vi "Format InstanceNetworkInterfaceSetItemType_LVXML_Loop.vi"(8 "error in (no error)":errorcluster, 10 "Siblings in 3":T2(array[cluster]), 11 "AWS_EC2 in":refnum<class "AWS_EC2.lvclass">) -> (0 "error out":errorcluster, 2 "Array":T3[](array[typedef]), 3 "AWS_EC2 out":refnum<class "AWS_EC2.lvclass">)   [LabVIEW 2014, in "AWS_EC2.lvlib" / "AWS_EC2.lvclass"]
uses:
  AWS_EC2.lvclass
  EC2 Datatypes/InstanceNetworkInterfaceSetItemType.ctl
  EC2 Datatypes/GroupItemTypeSet.ctl
  EC2 Datatypes/GroupItemType.ctl
  EC2 Datatypes/InstanceNetworkInterfaceAttachmentType.ctl
  EC2 Datatypes/InstanceNetworkInterfaceAssociationType.ctl
  EC2 Datatypes/InstancePrivateIpAddressesSetItemType.ctl
  lv-xml-parser/r0/trunk/VI Source/EventType.ctl
  AWS_EC2.lvlib
  lv-xml-parser/r0/trunk/VI Source/LV XML Parser.lvlib
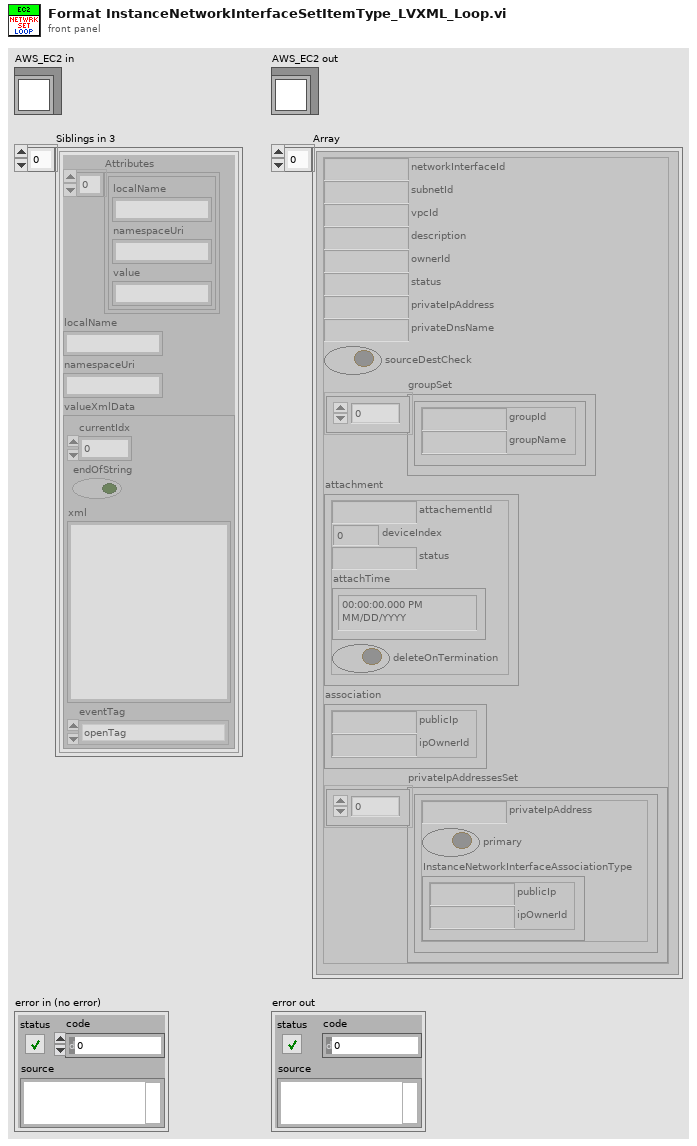
[diagram p1: front panel]
types:
  T1 = typedef "LV XML Parser.lvlib/EventType.ctl" = enum16{"openTag", "endOpenTag", "closeTag", "comment", "endComment", "endOfFile", "attribute", "startXml", "selfClosingTag"}
  T2 = cluster{"Attributes":cluster{"localName":string, "namespaceUri":string, "value":string}[], "localName":string, "namespaceUri":string, "valueXmlData":cluster{"currentIdx":i32, "endOfString":bool, "xml":string, "eventTag":T1}}[]
  T3 = typedef "AWS_EC2.lvlib/InstanceNetworkInterfaceSetItemType.ctl" = cluster{"networkInterfaceId":string, "subnetId":string, "vpcId":string, "description":string, "ownerId":string, "status":string, "privateIpAddress":string, "privateDnsName":string, "sourceDestCheck":bool, "groupSet":T4, "attachment":T6, "association":T7, "privateIpAddressesSet":T8[]}
  T4 = typedef "AWS_EC2.lvlib/GroupItemTypeSet.ctl" = T5[]
  T5 = typedef "AWS_EC2.lvlib/GroupItemType.ctl" = cluster{"groupId":string, "groupName":string}
  T6 = typedef "AWS_EC2.lvlib/InstanceNetworkInterfaceAttachmentType.ctl" = cluster{"attachementId":string, "deviceIndex":i32, "status":string, "attachTime":timestamp, "deleteOnTermination":bool}
  T7 = typedef "AWS_EC2.lvlib/InstanceNetworkInterfaceAssociationType.ctl" = cluster{"publicIp":string, "ipOwnerId":string}
  T8 = typedef "AWS_EC2.lvlib/InstancePrivateIpAddressesSetItemType.ctl" = cluster{"privateIpAddress":string, "primary":bool, "InstanceNetworkInterfaceAssociationType":T7}
  T9 = cluster{"Attributes":cluster{"localName":string, "namespaceUri":string, "value":string}[], "localName":string, "namespaceUri":string, "valueXmlData":cluster{"currentIdx":i32, "endOfString":bool, "xml":string, "eventTag":T1}}
  T10 = cluster{"currentIdx":i32, "endOfString":bool, "xml":string, "eventTag":T1}
  T11 = cluster{"namespaceUri":string, "localName":string}
  T12 = cluster{"Attributes":cluster{"localName":string, "namespaceUri":string, "value":string}[], "localName":string, "namespaceUri":string, "valueXmlData":cluster{"currentIdx":i64, "endOfString":bool, "xml":string, "eventTag":T1}}[]
  T13 = cluster{"currentIdx":i64, "endOfString":bool, "xml":string, "eventTag":T1}
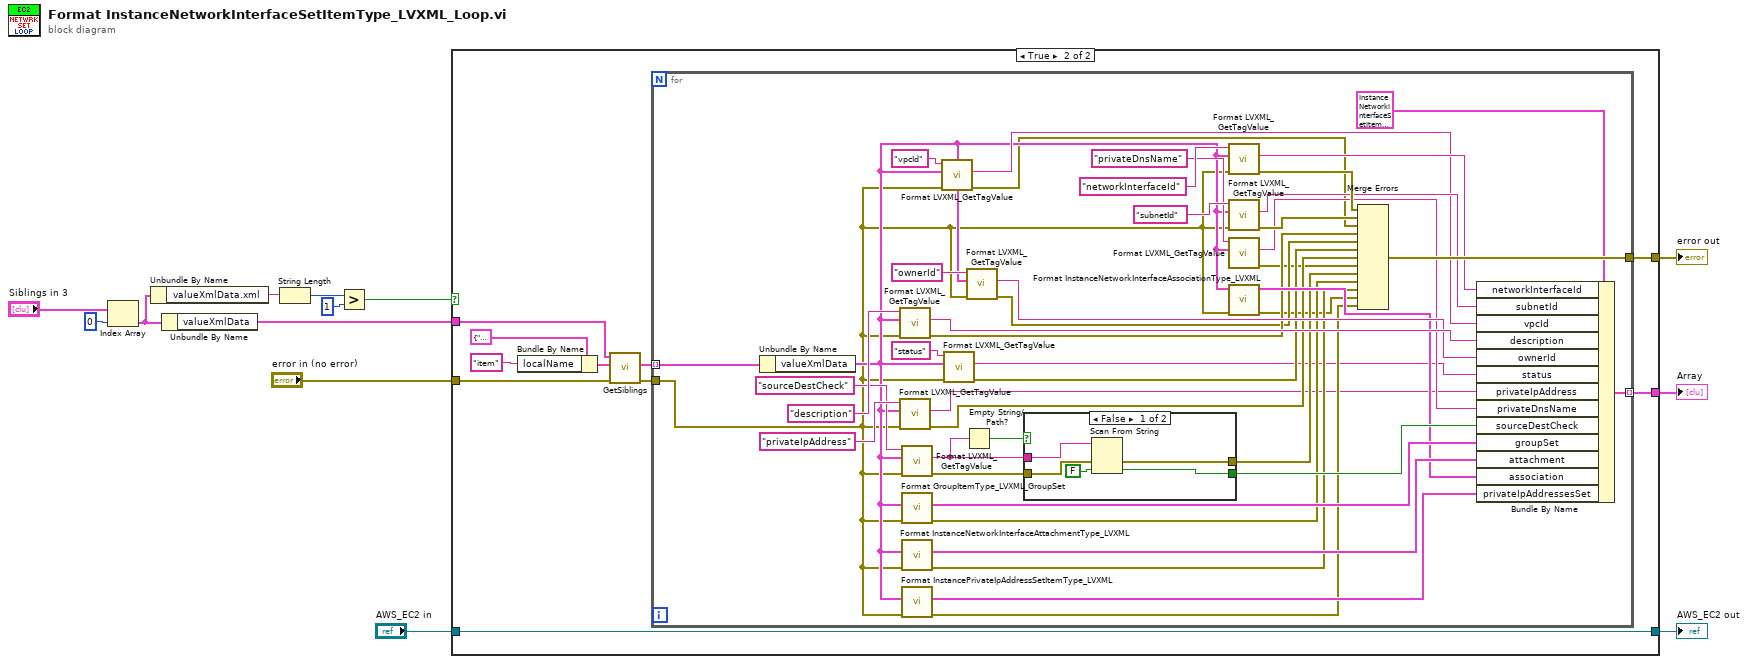
[diagram p0: block diagram]
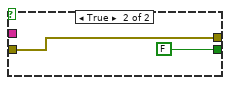
[diagram p3: hidden frame]
diagram:
  n1 = Index Array(array="Siblings in 3", index=0) -> (element=w3:T9)
  n2 = Unbundle By Name(w3) -> ("valueXmlData.xml"=w4:string)
  n3 = Unbundle By Name(w3) -> ("valueXmlData"=w5:T10)
  n4 = String Length(string=w4) -> (length=w8:i32)
  n5 = Greater?(x=w8, y=1) -> (0:w6:bool)
  n6 = case shown="True" w6 {
    tunnel: [w15 w24] -> w12
    tunnel: "error in (no error)" -> [w15 w19]
    tunnel: w5 -> [_ w18]
    tunnel: "AWS_EC2 in" -> [w14 w17]
    tunnel: [w14 w17] -> w1
    tunnel: [_ w16] -> w13
    frame False {
    }
    frame True {
      n7 = Bundle By Name(cluster=T11 {"namespaceUri"="", "localName"=""} ("limitToTag"), "localName"="item" ("Tag name")) -> (w21:T11)
      n8 = call "GetSiblings.vi"("error in (no error)"=w19, "limitToTag"=w21, "xmlData"=w18) -> ("error out"=w25:errorcluster, "Siblings"=w22:T12)  [unwired: 7 in]
      n9 = for {
        tunnel: w22 -> [w69] mode=indexing
        tunnel: [w68] -> w24
        tunnel: w25 -> [w40]
        tunnel: [w62] -> w16 mode=indexing
        n10 = Unbundle By Name(w69) -> ("valueXmlData"=w41:T13)
        n11 = call "Format LVXML_GetTagValue.vi"("error in (no error)"=w40, "xmlDataIn"=w41, "Tag name"="description") -> ("error out"=w37:errorcluster, "Value"=w56:string)  [unwired: 6 in, 1 out]
        n12 = call "Format LVXML_GetTagValue.vi"("error in (no error)"=w40, "xmlDataIn"=w41, "Tag name"="privateIpAddress") -> ("error out"=w34:errorcluster, "Value"=w27:string)  [unwired: 6 in, 1 out]
        n13 = call "Format LVXML_GetTagValue.vi"("error in (no error)"=w40, "xmlDataIn"=w41, "Tag name"="sourceDestCheck") -> ("error out"=w47:errorcluster, "Value"=w48:string)  [unwired: 6 in, 1 out]
        n14 = call "Format GroupItemType_LVXML_GroupSet.vi"("error in (no error)"=w40, "valueXmlData"=w41) -> ("error out"=w31:errorcluster, "Array"=w44:T5[])  [unwired: 7 in, 1 out]
        n15 = call "Format InstanceNetworkInterfaceAttachmentType_LVXML.vi"("error in (no error)"=w40, "xmlData in"=w41) -> ("error out"=w30:errorcluster, "InstanceNetworkInterfaceAttachmentType"=w43:T6)  [unwired: 7 in, 1 out]
        n16 = call "Format InstancePrivateIpAddressSetItemType_LVXML.vi"("error in (no error)"=w40, "valueXmlData 3"=w41) -> ("error out"=w28:errorcluster, "Array"=w39:T8[])  [unwired: 7 in, 1 out]
        n17 = call "Format LVXML_GetTagValue.vi"("error in (no error)"=w40, "xmlDataIn"=w41, "Tag name"="vpcId") -> ("error out"=w38:errorcluster, "Value"=w58:string)  [unwired: 6 in, 1 out]
        n18 = call "Format LVXML_GetTagValue.vi"("error in (no error)"=w40, "xmlDataIn"=w41, "Tag name"="status") -> ("error out"=w35:errorcluster, "Value"=w26:string)  [unwired: 6 in, 1 out]
        n19 = Empty String/Path?(string/path=w48) -> (empty?=w49:bool)
        n20 = call "Format LVXML_GetTagValue.vi"("error in (no error)"=w40, "xmlDataIn"=w41, "Tag name"="ownerId") -> ("error out"=w36:errorcluster, "Value"=w54:string)  [unwired: 6 in, 1 out]
        n21 = case shown="False" w49 {
          tunnel: [w74 w76] -> w32
          tunnel: [w73 FALSE] -> w45
          tunnel: w47 -> [w71 w76]
          tunnel: w48 -> [w70 _]
          frame False {
            n22 = Scan From String(input string=w70, error in=w71, default 1=FALSE) -> (error out=w74:errorcluster, output 1=w73:bool)  [unwired: 2 in, 2 out]
          }
          frame True {
          }
        }
        n23 = call "Format LVXML_GetTagValue.vi"("error in (no error)"=w40, "xmlDataIn"=w41, "Tag name"="networkInterfaceId") -> ("error out"=w65:errorcluster, "Value"=w61:string)  [unwired: 6 in, 1 out]
        n24 = call "Format LVXML_GetTagValue.vi"("error in (no error)"=w40, "xmlDataIn"=w41, "Tag name"="subnetId") -> ("error out"=w64:errorcluster, "Value"=w60:string)  [unwired: 6 in, 1 out]
        n25 = call "Format LVXML_GetTagValue.vi"("xmlDataIn"=w41, "Tag name"="privateDnsName") -> ("error out"=w33:errorcluster, "Value"=w50:string)  [unwired: 7 in, 1 out]
        n26 = call "Format InstanceNetworkInterfaceAssociationType_LVXML.vi"("error in (no error)"=w40, "xmlData in"=w41) -> ("error out"=w29:errorcluster, "InstanceNetworkInterfaceAssociationType"=w42:T7)  [unwired: 8 in]
        n27 = Merge Errors(w65, w64, w38, w37, w36, w35, w34, w33, w32, w31, w30, w29, w28) -> (w68:errorcluster)
        n28 = Bundle By Name(cluster=T3 {"networkInterfaceId"="", "subnetId"="", "vpcId"="", "description"="", "ownerId"="", "status"="", "privateIpAddress"="", "privateDnsName"="", "sourceDestCheck"=FALSE, "groupSet"=[], "attachment"={"attachementId"="", "deviceIndex"=0, "status"="", "attachTime"=timestamp(0 s since 1904-01-01), "deleteOnTermination"=FALSE}, "association"={"publicIp"="", "ipOwnerId"=""}, "privateIpAddressesSet"=[]} ("InstanceNetworkInterfaceSetItemType"), "networkInterfaceId"=w61, "subnetId"=w60, "vpcId"=w58, "description"=w56, "ownerId"=w54, "status"=w26, "privateIpAddress"=w27, "privateDnsName"=w50, "sourceDestCheck"=w45, "groupSet"=w44, "attachment"=w43, "association"=w42, "privateIpAddressesSet"=w39) -> (w62:T3)
      }
    }
  }
  "Array" <- w13
  "error out" <- w12
  "AWS_EC2 out" <- w1
